vi "populate_config_combos.vi"(7 "configurations":T1[](array[typedef]), 8 "error in (no error)":errorcluster, 9 "plug-in path refs":refnum<vi>[](array[refnum]), 10 "combo control refs":refnum<vi>[](array[refnum]), 11 "GenericPlugin in":refnum<class "GenericComponent.lvclass">) -> (0 "error out":errorcluster, 3 "GenericPlugin out":refnum<class "GenericComponent.lvclass">)   [LabVIEW 2010, in "GenericComponent.lvclass"]
doc: "This VI populates i) combo boxes with the names of config files and ii) path controls with plug-in class paths."
uses:
  GenericComponent.lvclass
  clusters/plugin_specification.ctl
  <vilib>/regexp/Match Regular Expression.xnode
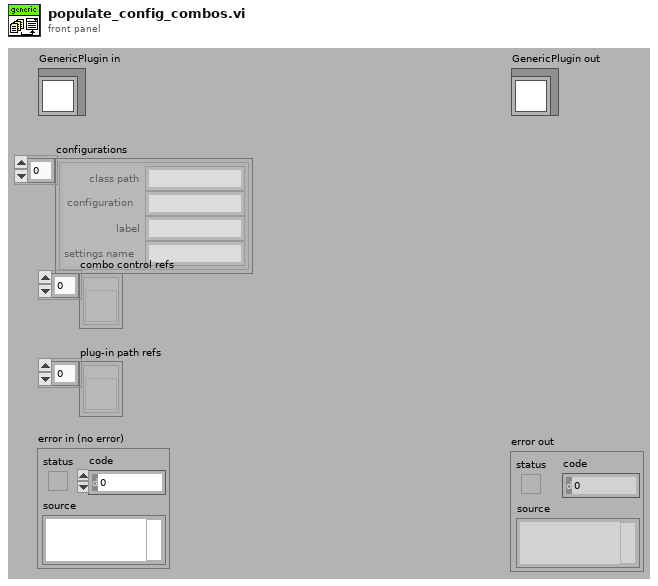
[diagram p1: front panel]
types:
  T1 = typedef "plugin_specification.ctl" = cluster{"class path":string, "configuration":string, "label":string, "settings name":string}
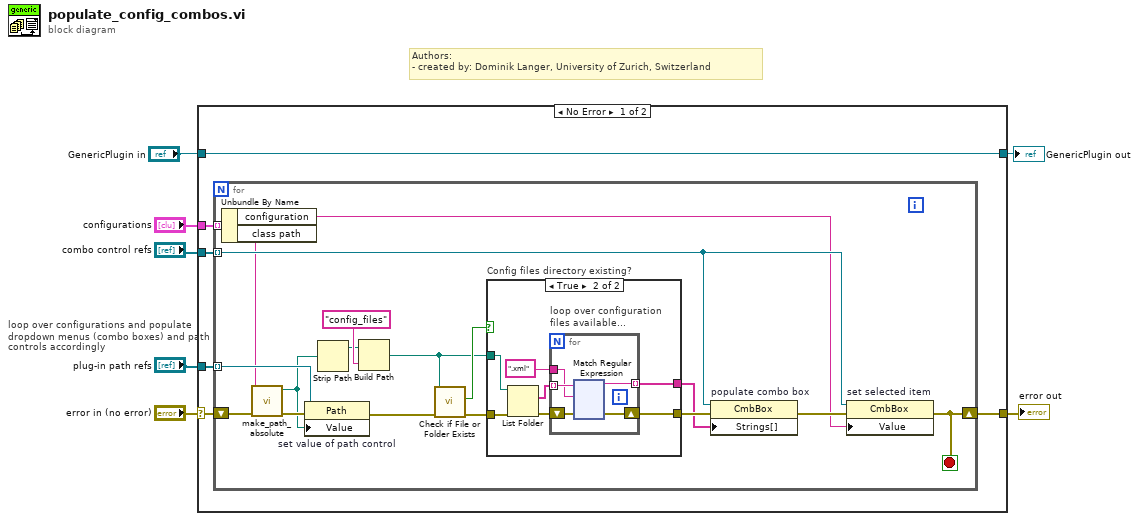
[diagram p0: block diagram]
diagram:
  # "Authors: \n- created by: Dominik Langer, University of Zurich, Switzerland"
  n1 = case shown="No Error" "error in (no error)" {
    selector: "error in (no error)" -> [w12 w157]
    tunnel: [w11 w157] -> w6
    tunnel: [w13 w156] -> w4
    tunnel: "GenericPlugin in" -> [w13 w156]
    tunnel: "configurations" -> [w10 _]
    tunnel: "combo control refs" -> [w9 _]
    tunnel: "plug-in path refs" -> [w8 _]
    frame No Error {
      n2 = for "loop over configurations and populate dropdown menus (combo boxes) and path controls accordingly" {
        tunnel: w10 -> [w27] mode=indexing
        tunnel: w9 -> [w28] mode=indexing
        tunnel: w8 -> [w25] mode=indexing
        shift-right: [w22] -> w11
        shift-left: w12 -> [w17]
        stop <- w22 stop-if-true
        n3 = Unbundle By Name(w27) -> ("configuration"=w26:string, "class path"=w14:string)
        n4 = call "make_path_absolute.vi"("error in (no error)"=w17, "relative path"=w14) -> ("error out"=w16:errorcluster, "absolute path"=w15:path)  [unwired: 8 in]
        n5 = property on="set value of path control" class="Path"(reference=w25, error in=w16, "Value"=w15) -> (error out=w21:errorcluster)  [unwired: 1 out]
        n6 = Strip Path(path=w15) -> (stripped path=w23:path)  [unwired: 1 out]
        n7 = Build Path(base path=w23, name or relative path="config_files") -> (appended path=w18:path)
        n8 = call <vilib>:"Check if File or Folder Exists.vi"("error in (no error)"=w21, "path"=w18) -> ("error out"=w20:errorcluster, "file or folder exists?"=w19:bool)  [unwired: 8 out]
        n9 = case "Config files directory existing?" shown="True" w19 {
          tunnel: [w32 w39] -> w31
          tunnel: [_ w38] -> w30
          tunnel: w20 -> [w32 w34]
          tunnel: w18 -> [_ w33]
          frame False {
          }
          frame True {
            n10 = List Folder(path=w33, error in=w34) -> (filenames=w35:string[], error out=w36:errorcluster)  [unwired: 4 out]
            n11 = for "loop over configuration files available..." {
              tunnel: w35 -> [w44] mode=indexing
              tunnel: [w43] -> w38 mode=indexing
              tunnel: ".xml" ("regular expression") -> [w41]
              shift-right: [w40] -> w39
              shift-left: w36 -> [w42]
              n12 = xnode "Match Regular Expression"("input string"=w44, "regular expression"=w41, "error in"=w42) -> ("before match"=w43:string, "error out"=w40:errorcluster)  [unwired: 1 in, 5 out]
            }
          }
        }
        n13 = property on="populate combo box" class="CmbBox"(reference=w28, error in=w31, "Strings[]"=w30) -> (error out=w29:errorcluster)  [unwired: 1 out]
        n14 = property on="set selected item" class="CmbBox"(reference=w28, error in=w29, "Value"=w26) -> (error out=w22:errorcluster)  [unwired: 1 out]
      }
    }
    frame Error {
    }
  }
  "error out" <- w6
  "GenericPlugin out" <- w4
